vi "Change DataFolders File Name_PM.vi"(6 "error in (no error)":errorcluster, 7 "Value":path, 8 "ROI Name":string, 9 "Value 2":u16, 10 "Strings []":string[](array[string])) -> (4 "error out":errorcluster)   [LabVIEW 2019]
uses:
  ROI/Controls/ROI_List_Action.ctl
  Analysis/Controls/Parttern Match/Analysis_PatternMatch_Parameter.ctl
  Process/Controls/Process_Setting.ctl
  Analysis/Controls/Analysis_Setting.ctl
  Controls/Vision_DataEntry.ctl
  Analysis/Controls/V_Analysis_Type.ctl
  Ctrl/VisionProcessName.ctl
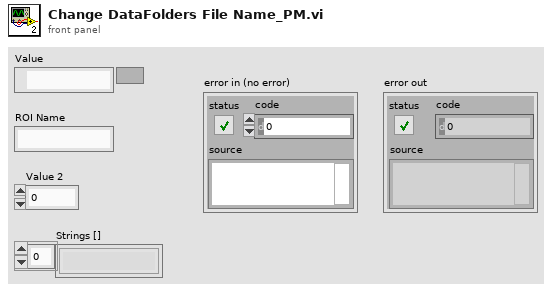
[diagram p1: front panel]
types:
  T1 = typedef "ROI_List_Action.ctl" = enum16{"Init", "Add ROI", "Delete ROI", "Get All ROI", "Get Specific ROI", "Set Analysis Setting", "Set Process Setting", "Replace All Entries", "ROIEntryBackup", "ROIEntryBackupClear", "ROIEntryReturn"}
  T2 = typedef "Vision_DataEntry.ctl" = cluster{"vROIName":string, "vROIContour":cluster{"Contour Type":u32, "ROI Type":u32, "Points":i32[]}, "ProcessSetting":T3[], "Analysis_Setting":T5}
  T3 = typedef "Process_Setting.ctl" = cluster{"Enum_PreProcess":T4, "Parameter":string}
  T4 = typedef "VisionProcessName.ctl" = enum16{"*CamParameter*", "CamAttributes", "*Preprocess*", "CG_Brightness", "C_Plane Extraction", "C_Threshold", "G_Lookup Table", "G_Threshold"}
  T5 = typedef "Analysis_Setting.ctl" = cluster{"PreProcess":T6, "Parameter":string}
  T6 = typedef "V_Analysis_Type.ctl" = enum16{"None", "C_Color Pattern Matching", "G_PatternMatching", "G_ShapeDectect", "G_GeometricMatch", "B_Area Check"}
  T7 = typedef "Analysis_PatternMatch_Parameter.ctl" = cluster{"Algorithm":i32, "Match Parameters":cluster{"Number of Matches Requested":i32, "Minimum Match Score":sgl, "Angle Ranges":cluster{"Start Angle":sgl, "End Angle":sgl}[]}, "ROI Descriptor":T8, "Advanced Options":cluster{"Item":u16, "Value":dbl}[], "Template path":string, "XOffset":i32, "YOffset":i32}
  T8 = typedef "ROI Descriptor" = cluster{"Global Rectangle":i32[], "Contours":cluster{"ID":enum32{"External", "Internal"}, "Type":u32, "Coordinates":i32[]}[]}
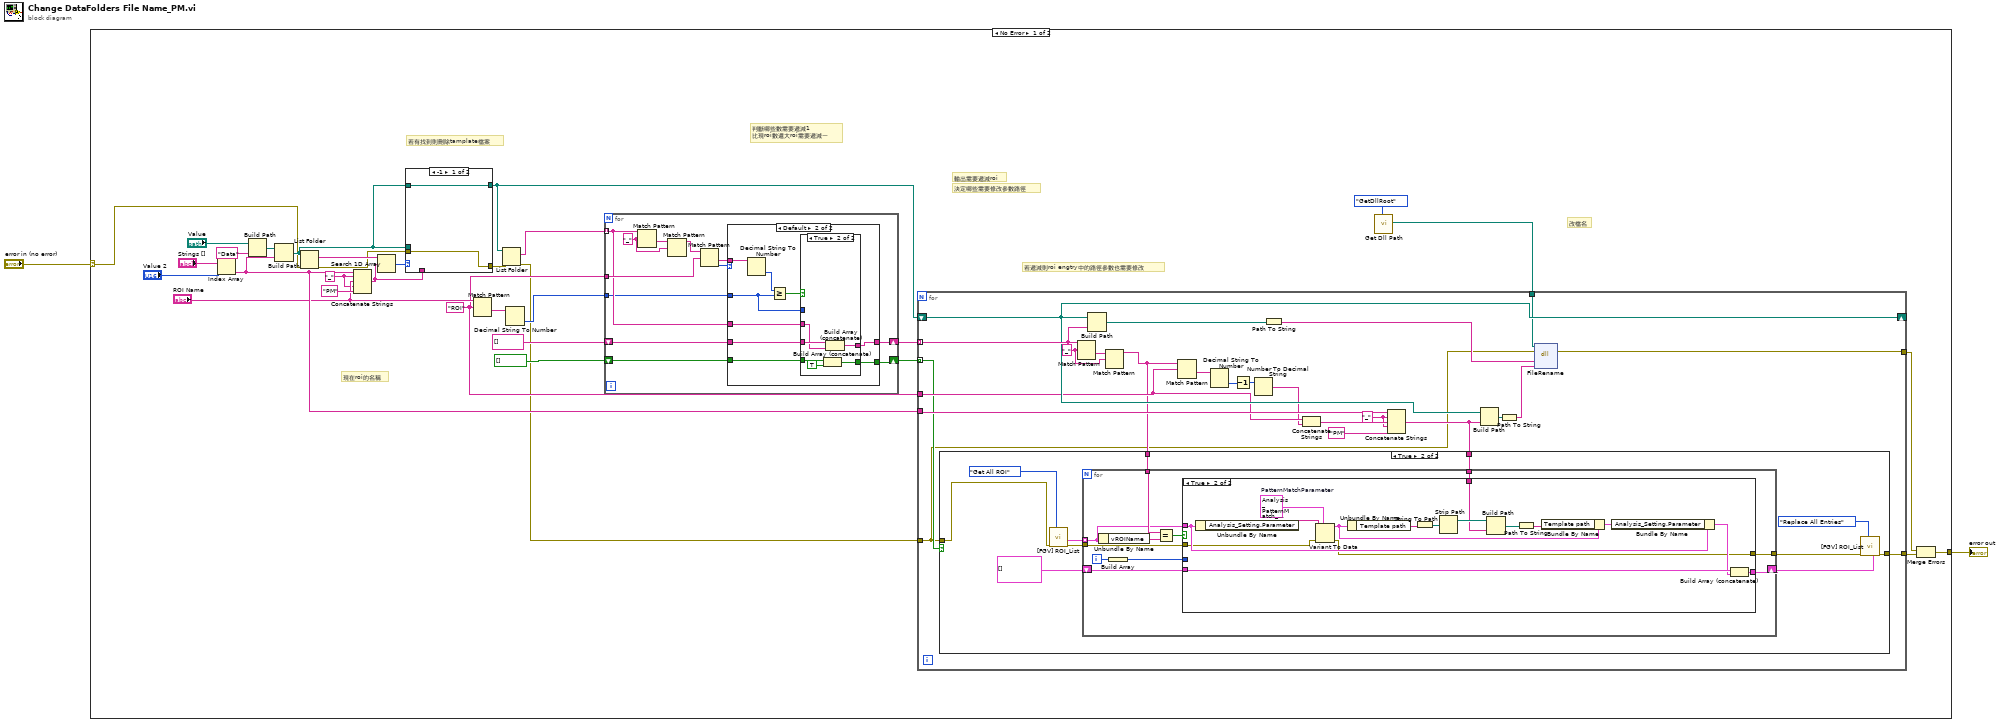
[diagram p0: block diagram]
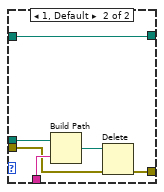
[diagram p2: hidden frame]
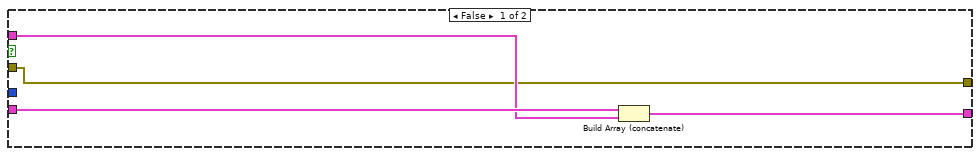
[diagram p4: hidden frame]
diagram:
  n1 = case shown="No Error" "error in (no error)" {
    selector: "error in (no error)" -> [w9 w140]
    tunnel: [w6 w140] -> w1
    frame No Error {
      w19 = "ROI" ("regular expression")
      w24 = "_" ("string")
      # "改檔名"
      # "決定哪些需要修改參數路徑"
      # "若遞減則roi engtry中的路徑參數也需要修改"
      # "輸出需要遞減roi"
      # "判斷哪些數需要遞減1\n比現roi數還大roi需要遞減一"
      # "若有找到則刪除tamplate檔案"
      # "現在roi的名稱"
      n2 = Index Array(array="Strings []", index="Value 2") -> (element=w26:string)
      n3 = Build Path(base path="Value", name or relative path="Data") -> (appended path=w30:path)
      n4 = Build Path(base path=w30, name or relative path=w26) -> (appended path=w16:path)
      n5 = List Folder(path=w16, error in=w9) -> (filenames=w17:string[], error out=w10:errorcluster)  [unwired: 2 in, 2 out]
      n6 = Concatenate Strings(w26, w24, "ROI Name", w24, "PM") -> (w33:string)
      n7 = Search 1D Array(1D array=w17, element=w33) -> (index of element=w18:i32)  [unwired: 1 in]
      n8 = case shown="-1" w18 {
        tunnel: w16 -> [_ w41]
        tunnel: w33 -> [_ w40]
        tunnel: [w35 w38] -> w15
        tunnel: w16 -> [w35 w38]
        tunnel: [w34 w37] -> w11
        tunnel: w10 -> [w34 w36]
        frame -1 {
        }
        frame 1, Default {
          n9 = Build Path(base path=w41, name or relative path=w40) -> (appended path=w39:path)
          n10 = Delete(path (use dialog)=w39, error in=w36) -> (error out=w37:errorcluster)  [unwired: 3 in, 2 out]
        }
      }
      n11 = Match Pattern(string="ROI Name", regular expression=w19) -> (after substring=w23:string)  [unwired: 1 in, 3 out]
      n12 = List Folder(path=w15, error in=w11) -> (filenames=w14:string[], error out=w5:errorcluster)  [unwired: 2 in, 2 out]
      n13 = Decimal String To Number(string=w23) -> (number=w22:i32)  [unwired: 2 in, 1 out]
      n14 = for {
        tunnel: w14 -> [w116] mode=indexing
        tunnel: w19 -> [w118]
        tunnel: w22 -> [w112]
        shift-right: [w114] -> w20
        shift-left: string[] [] -> [w115]
        shift-right: [w110] -> w12
        shift-left: bool[] [] -> [w111]
        w119 = "_" ("regular expression")
        n15 = Match Pattern(string=w116, regular expression=w119) -> (after substring=w120:string)  [unwired: 1 in, 3 out]
        n16 = Match Pattern(string=w120, regular expression=w119) -> (before substring=w113:string)  [unwired: 1 in, 3 out]
        n17 = Match Pattern(string=w113, regular expression=w118) -> (after substring=w117:string, offset past match=w109:i32)  [unwired: 1 in, 2 out]
        n18 = case shown="Default" w109 {
          tunnel: w117 -> [_ w131]
          tunnel: w116 -> [_ w128]
          tunnel: w115 -> [w122 w127]
          tunnel: [w122 w126] -> w114
          tunnel: w112 -> [_ w125]
          tunnel: w111 -> [w121 w124]
          tunnel: [w121 w123] -> w110
          frame -1 {
          }
          frame Default {
            n19 = Decimal String To Number(string=w131) -> (number=w130:i32)  [unwired: 2 in, 1 out]
            n20 = Greater Or Equal?(x=w130, y=w125) -> (x >= y?=w129:bool)
            n21 = case shown="True" w129 {
              tunnel: w128 -> [_ w137]
              tunnel: w127 -> [w133 w139]
              tunnel: [w133 w138] -> w126
              tunnel: w125 -> [_ _]
              tunnel: w124 -> [w132 w136]
              tunnel: [w132 w135] -> w123
              frame False {
              }
              frame True {
                n22 = Build Array (concatenate)(w136, TRUE) -> (w135:bool[])
                n23 = Build Array (concatenate)(w139, w137) -> (w138:string[])
              }
            }
          }
        }
      }
      n24 = call "Get Dll Path.vi"("Action"=enum16{"WriteDllRoot", "GetDllRoot"}."GetDllRoot") -> ("Dll Root Path"=w3:path)  [unwired: 10 in]
      n25 = for {
        tunnel: w20 -> [w60] mode=indexing
        tunnel: w19 -> [w53]
        shift-right: [w56] -> _
        shift-left: w15 -> [w56]
        tunnel: w26 -> [w57]
        tunnel: [w48] -> w7
        tunnel: w12 -> [w45] mode=indexing
        tunnel: [w44] -> w8
        tunnel: w5 -> [w43]
        tunnel: w3 -> [w42]
        w50 = "_" ("string")
        w64 = "_" ("regular expression")
        n26 = Match Pattern(string=w60, regular expression=w64) -> (after substring=w63:string)  [unwired: 1 in, 3 out]
        n27 = Build Path(base path=w56, name or relative path=w60) -> (appended path=w59:path)
        n28 = Match Pattern(string=w63, regular expression=w64) -> (before substring=w47:string)  [unwired: 1 in, 3 out]
        n29 = Match Pattern(string=w47, regular expression=w53) -> (after substring=w65:string)  [unwired: 1 in, 3 out]
        n30 = Decimal String To Number(string=w65) -> (number=w62:i32)  [unwired: 2 in, 1 out]
        n31 = Decrement(x=w62) -> (x-1=w61:i32)
        n32 = Number To Decimal String(number=w61) -> (decimal integer string=w52:string)  [unwired: 1 in]
        n33 = Path To String(path=w59) -> (string=w58:string)
        n34 = Concatenate Strings(w53, w52) -> (w51:string)
        n35 = Concatenate Strings(w57, w50, w51, w50, "PM" ("string")) -> (w46:string)
        n36 = case shown="True" w45 {
          tunnel: w47 -> [_ w76]
          tunnel: w46 -> [_ w75]
          tunnel: [w66 w70] -> w44
          tunnel: w43 -> [w66 w67]
          frame False {
          }
          frame True {
            n37 = call "[FGV] ROI_List.vi"("Action"=ROI_List_Action."Get All ROI", "error in (no error)"=w67) -> ("error out"=w68:errorcluster, "All ROI"=w77:T2[])  [unwired: 7 in, 1 out]
            n38 = for {
              tunnel: w77 -> [w83] mode=indexing
              tunnel: w76 -> [w87]
              tunnel: w75 -> [w82]
              shift-right: [w80] -> w71
              shift-left: T2[] [] -> [w81]
              tunnel: [w79] -> w69
              tunnel: w68 -> [w78]
              i -> [w85]
              n39 = Unbundle By Name(w83) -> ("vROIName"=w88:string)
              n40 = Build Array(w85) -> (w84:i32[])
              n41 = Equal?(x=w87, y=w88) -> (x = y?=w86:bool)
              n42 = case shown="True" w86 {
                tunnel: w84 -> [_ _]
                tunnel: w83 -> [w91 w99]
                tunnel: w82 -> [_ w103]
                tunnel: w81 -> [w92 w97]
                tunnel: [w90 w95] -> w80
                tunnel: [w89 w94] -> w79
                tunnel: w78 -> [w89 w93]
                frame False {
                  n43 = Build Array (concatenate)(w92, w91) -> (w90:T2[])
                }
                frame True {
                  w107 = T7 {"Algorithm"=2, "Match Parameters"={"Number of Matches Requested"=1, "Minimum Match Score"=750.0, "Angle Ranges"=[]}, "ROI Descriptor"={"Global Rectangle"=[], "Contours"=[]}, "Advanced Options"=[{"Item"=1, "Value"=1.0}, {"Item"=103, "Value"=1.0}], "Template path"="", "XOffset"=0, "YOffset"=0}  # PatternMatchParameter
                  n44 = Unbundle By Name(w99) -> ("Analysis_Setting.Parameter"=w108:string)
                  n45 = Variant To Data(error in=w93, type=w107, Variant=w108) -> (data=w101:T7, error out=w94:errorcluster)
                  n46 = Unbundle By Name(w101) -> ("Template path"=w106:string)
                  n47 = String To Path(string=w106) -> (path=w105:path)
                  n48 = Strip Path(path=w105) -> (stripped path=w104:path)  [unwired: 1 out]
                  n49 = Build Path(base path=w104, name or relative path=w103) -> (appended path=w102:path)
                  n50 = Path To String(path=w102) -> (string=w100:string)
                  n51 = Bundle By Name(cluster=w101, "Template path"=w100) -> (w98:T7)
                  n52 = Bundle By Name(cluster=w99, "Analysis_Setting.Parameter"=w98) -> (w96:T2)
                  n53 = Build Array (concatenate)(w97, w96) -> (w95:T2[])
                }
              }
            }
            n54 = call "[FGV] ROI_List.vi"("ROIEntriesIn"=w71, "Action"=ROI_List_Action."Replace All Entries", "error in (no error)"=w69) -> ("error out"=w70:errorcluster)  [unwired: 6 in, 2 out]
          }
        }
        n55 = Build Path(base path=w56, name or relative path=w46) -> (appended path=w55:path)
        n56 = Path To String(path=w55) -> (string=w54:string)
        n57 = dll-call lib="C:/Users/user/Desktop/Smasoft/Project/iVision/20161003 Auto ROI/iVision_20161007_V1.6-3/SubVIs/File Name Dll/File Rename DLL.dll" fn="FileRename"(path in=w42, error in=w43, "OldName"=w58, "NewName"=w54) -> (error out=w48:errorcluster)  [unwired: 4 in, 1 out]
      }
      n58 = Merge Errors(w7, w8) -> (w6:errorcluster)
    }
    frame Error {
    }
  }
  "error out" <- w1
